vi "SayThisOnMIDAS.vi"(1 "String":string, 2 "Hostname (Optional)":string) -> (0 "error out":errorcluster)   [LabVIEW 2018, in "feGEM DataPacker.lvlib"]
uses:
  feGEM DataPacker.lvlib
  e72abe1d-083e-48c0-94c0-386f7adc7202.vi
  e72abe1d-083e-48c0-94c0-386f7adc7202.vi/adbfba35-8f5b-4c3e-9226-6d56bd61912d.vi
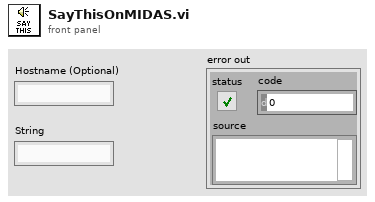
[diagram p1: front panel]
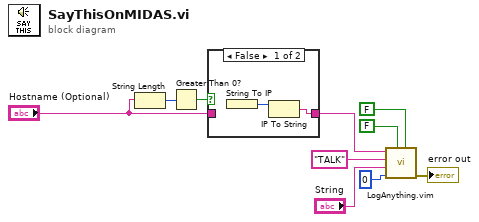
[diagram p0: block diagram]
diagram:
  n1 = String Length(string="Hostname (Optional)") -> (length=w10:i32)
  n2 = Greater Than 0?(x=w10) -> (x > 0?=w9:bool)
  n3 = case shown="False" w9 {
    tunnel: "Hostname (Optional)" -> [_ w13]
    tunnel: [w11 w13] -> w6
    frame False {
      n4 = String To IP() -> (0:w12:u32)  [unwired: 1 in]
      n5 = IP To String(2:w12) -> (0:w11:string)  [unwired: 1 in]
    }
    frame True {
    }
  }
  n6 = call "LogAnything.vim"("Skip ODB on the way to \nhistories (fast, but no ALARMS possible)"=FALSE ("Get Default History Period from MIDAS\n(optional)"), "FIFO (default = true)"=FALSE ("FIFO"), "Period to update history plots (seconds)\nUnset (65535) = Use MIDAS default in ODB\n0 = Record but do not put in histories"=0 ("Rate to update history plots"), "Array"="String", "Variable Name"="TALK" ("Equipment description"), "Category"=w6) -> ("error out"=→"error out":errorcluster)  [unwired: 5 in]
